vi "TAT_Start.vi"(8 "error In":errorcluster) -> ()   [LabVIEW 2017]
panel:
  out "Cycle Count":string
  out "Cycle Count":string
  out "BARCODE":string
  out "Cycle Status":string
  out "BARCODE":string
  out "RESULT":bool
  out "RESULT":bool
  out "VARIENT":string
  out "USER":string
  in  "ASS-Alarms":bool
  in  "T-Alarms":bool
  out "Cycle Status":string
  out "PLC RUN":bool
  out "DATE/TIME":string
  in  "stop":bool
  # "RBC ORVM- TRACEABILITY, SCANNING & BARCODE PRINTING"
  # "ASSEMBLY STATION"
  # "LEAKTEST STATION"
  # "Nm"
  # "KAPSE SONS ROBOTICS\n& AUTOMATION"
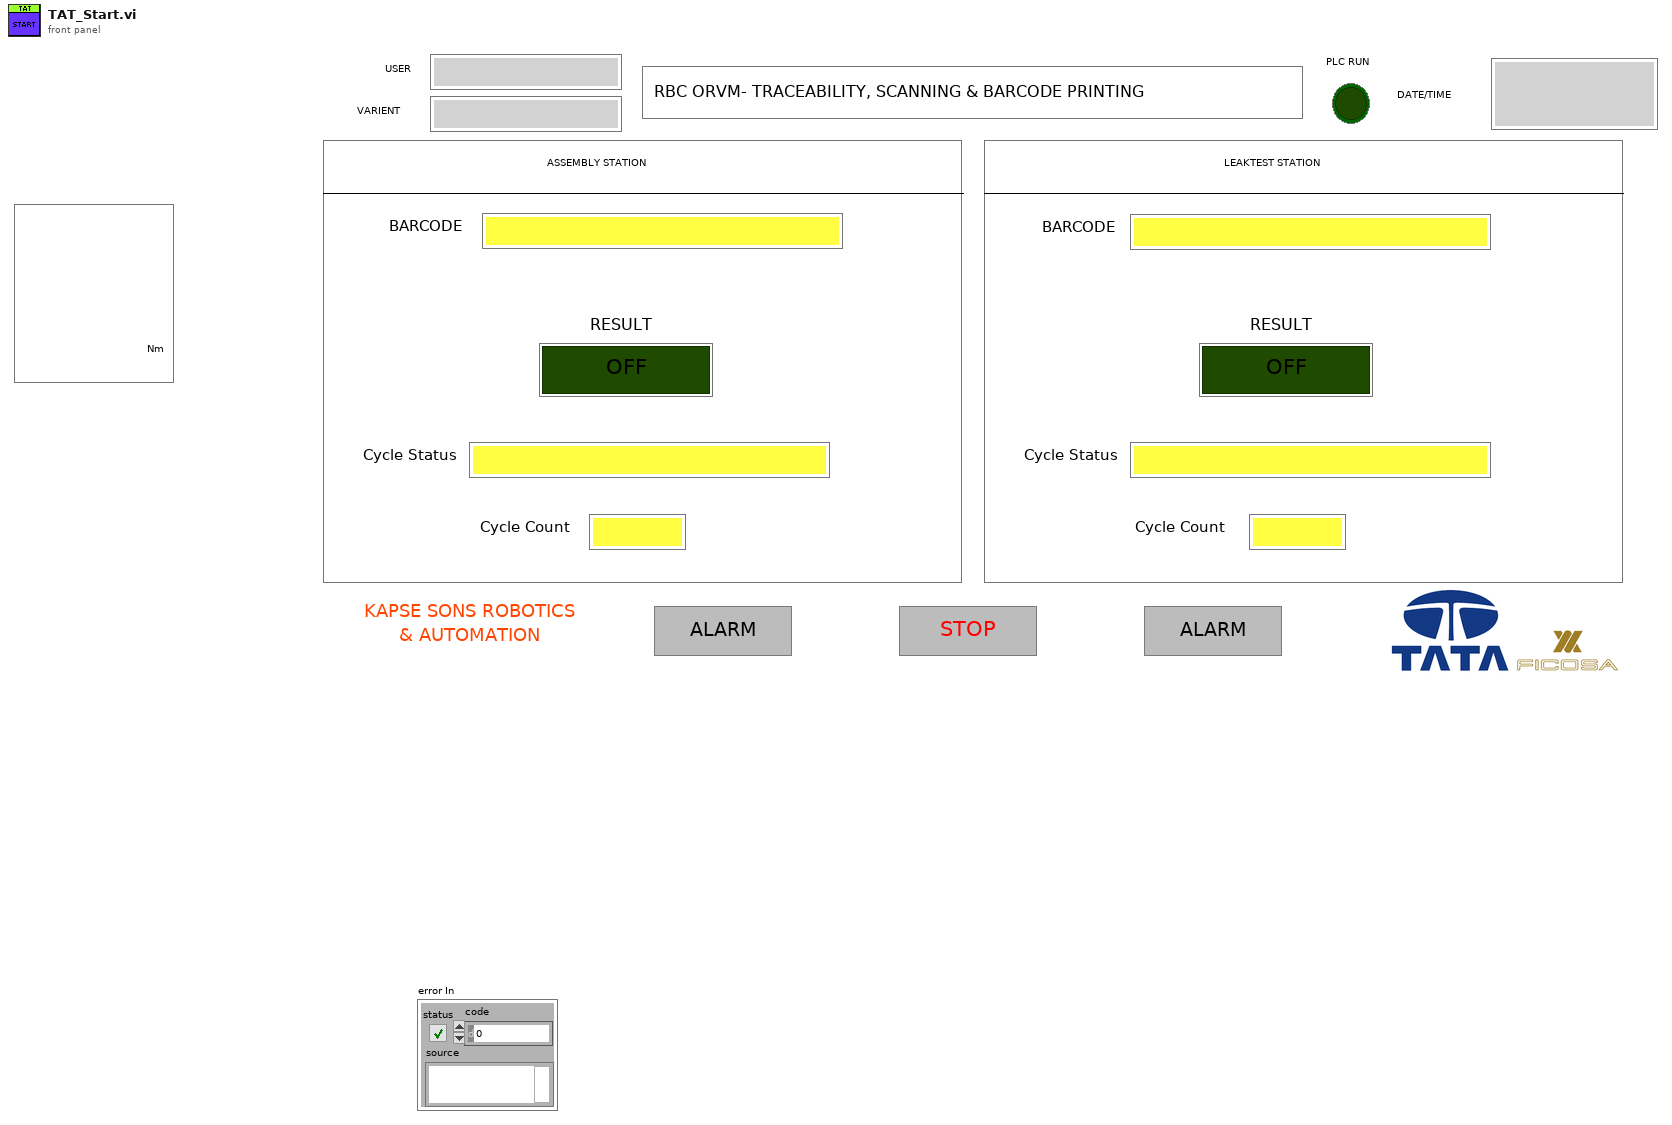
[diagram p1: front panel]
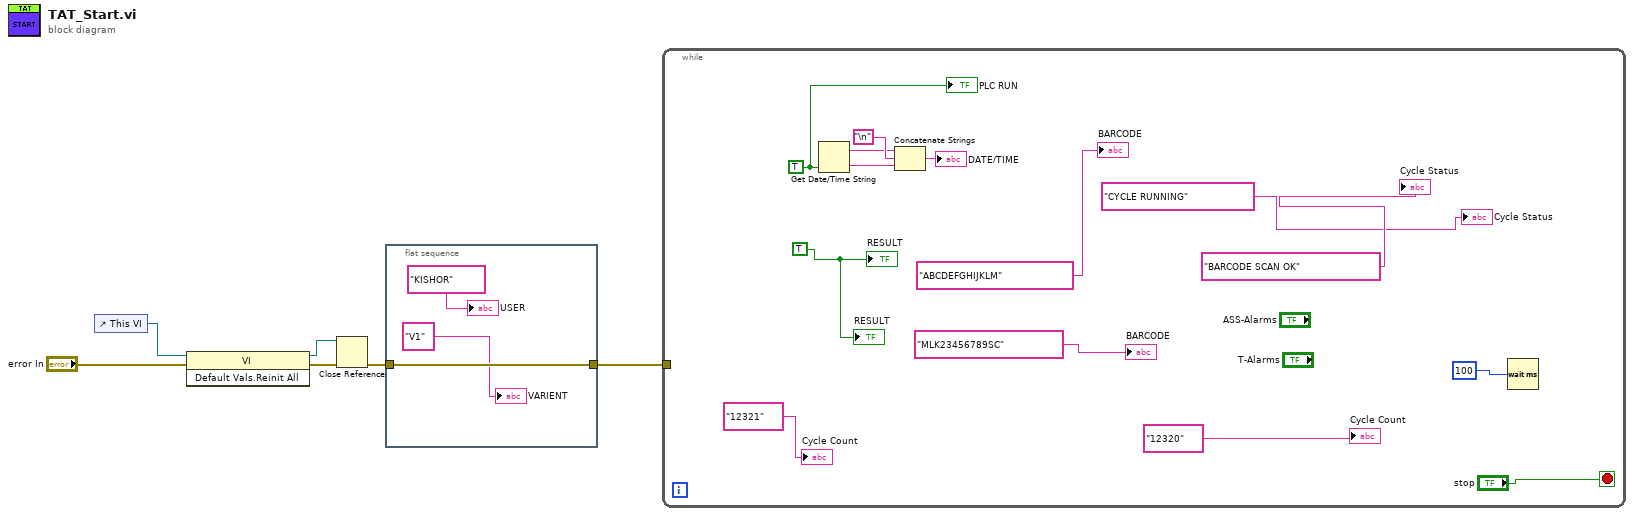
[diagram p0: block diagram]
diagram:
  n1 = control-ref of="This VI"() -> (w6:refnum<vi>)
  n2 = invoke class="VI" method="Default Vals.Reinit All"(reference=w6, error in="error In") -> (reference out=w3:refnum<vi>, error out=w4:errorcluster)  [unwired: 1 in, 1 out]
  n3 = Close Reference(reference=w3, error in (no error)=w4) -> (error out=w2:errorcluster)
  n4 = flat-sequence {
    tunnel: [w9] -> w1
    tunnel: w2 -> [w9]
    frame #0 {
      "USER" <- "KISHOR"
      "VARIENT" <- "V1"
    }
  }
  n5 = while {
    tunnel: w1 -> [_]
    stop <- "stop" stop-if-true
    w14 = TRUE ("want seconds? (F)")
    w13 = TRUE ("want seconds? (F)")
    n6 = Get Date/Time String(want seconds? (F)=w13) -> (date string=w19:string, time string=w18:string)  [unwired: 2 in]
    n7 = Concatenate Strings(w19, "\n", w18) -> (→"DATE/TIME":string)
    n8 = Wait (ms)(milliseconds to wait=u32 100) -> ()  [unwired: 1 out]
    "PLC RUN" <- w13
    "Cycle Status" <- "CYCLE RUNNING"
    "RESULT" <- w14
    "BARCODE" <- "ABCDEFGHIJKLM"
    "Cycle Status" <- "BARCODE SCAN OK"
    "BARCODE" <- "MLK23456789SC"
    "RESULT" <- w14
    "Cycle Count" <- "12321"
    "Cycle Count" <- "12320"
  }
